vi "S2_Motor_Set speed2015.vi"(8 "error in (no error)":errorcluster, 9 "baud rate (9600)":u32=9600, 11 "Resource Name 0":refnum<visa-resource-name>="COM4") -> (0 "Error Out":errorcluster={"status"=TRUE, "code"=-1073807343, "source"="VISA Write in Serial Communication for TL3T of VISA.vi"})   [LabVIEW 2012]
uses:
  2015myGlobal 1.vi
  <vilib>/Instr/_visa.llb/VISA Configure Serial Port (Instr).vi
panel:
  out "concatenated string":string="@0X2000,\r\n"
  out "重複次數":i32=5
  out "速度參數":i32=1600
  out "Step":i32=6400
  # "Step 1: Set parameters"
  # "Step 2: Setting Speed parameter"
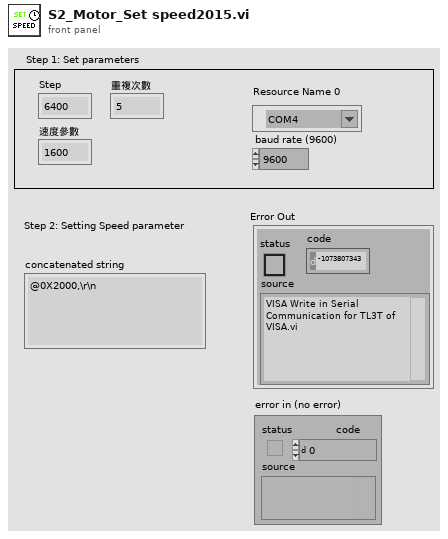
[diagram p1: front panel]
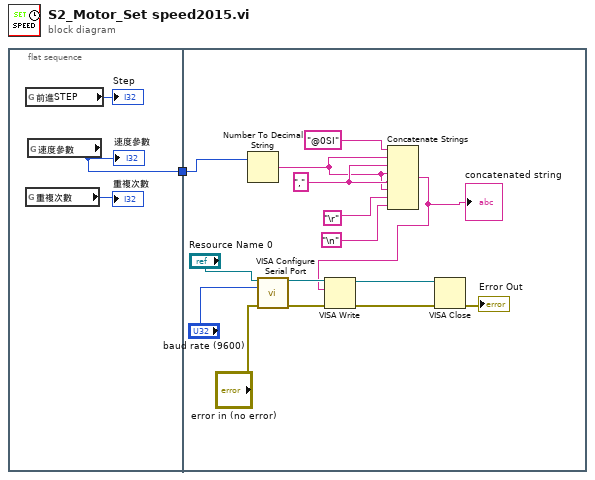
[diagram p0: block diagram]
diagram:
  n1 = flat-sequence {
    tunnel: [w2] -> w1
    tunnel: w1 -> [w9]
    frame #0 {
      n2 = global read "2015myGlobal 1.vi" "前進STEP"() -> (→"Step":i32)
      n3 = global read "2015myGlobal 1.vi" "重複次數"() -> (→"重複次數":i32)
      n4 = global read "2015myGlobal 1.vi" "速度參數"() -> (w2:i32)
      "速度參數" <- w2
    }
    frame #1 {
      w8 = "," ("string")
      n5 = Number To Decimal String(number=w9) -> (decimal integer string=w7:string)  [unwired: 1 in]
      n6 = call-poly "VISA Configure Serial Port"("VISA resource name"="Resource Name 0", "baud rate (9600)"="baud rate (9600)", "error in (no error)"="error in (no error)") -> ("VISA resource name out"=w16:refnum<visa-resource-name>, "error out"=w17:errorcluster)  [unwired: 11 in]
      n7 = Concatenate Strings("@0SI", w7, w8, w7, w8, w7, "\r", "\n") -> (w6:string)
      "concatenated string" <- w6
      n8 = VISA Write(VISA resource name=w16, write buffer=w6, error in (no error)=w17) -> (VISA resource name out=w18:refnum<visa-resource-name>, error out=w19:errorcluster)  [unwired: 1 out]
      n9 = VISA Close(VISA resource name=w18, error in (no error)=w19) -> (error out=→"Error Out":errorcluster)
    }
  }
